vi "Arbitrary Monitor Multigraph.vi"() -> ()   [LabVIEW 2022 SP3]
uses:
  <instrlib>/tio-labview/TIO Library/TIO Stream Open.vi
  <instrlib>/tio-labview/TIO Library/TIO RPC Send REQuest.vi
  <instrlib>/tio-labview/TIO Library/TIO RPC Parse Reply.vi
  <instrlib>/tio-labview/TIO Library/TIO RPC Parse Reply Error.vi
  <instrlib>/tio-labview/TIO Library/TIO Data Stream Parse timebase Info.vi
  <instrlib>/tio-labview/TIO Library/TIO Data Stream Parse pstream Info.vi
  <instrlib>/tio-labview/TIO Library/TIO Data Stream Parse dstream Info.vi
  <vilib>/Utility/High Resolution Relative Seconds.vi
  <instrlib>/tio-labview/TIO Library/TIO Serial Port Name Search.vi
  <instrlib>/tio-labview/TIO Library/TIO Stream Write.vi
  <instrlib>/tio-labview/TIO Library/TIO RPC Form Request.vi
  <instrlib>/tio-labview/TIO Library/TIO SLIP Serial Write.vi
  <instrlib>/tio-labview/TIO Library/TIO Form Packet.vi
  <instrlib>/tio-labview/TIO Library/TIO SLIP Encode.vi
  <instrlib>/tio-labview/TIO Library/TIO Serial Checksum CRC32.vi
  <vilib>/Utility/tcp.llb/UDP Multicast Open.vi
  <vilib>/Utility/tcp.llb/UDP Multicast Read-Write Open.vi
  <instrlib>/tio-labview/TIO Library/TIO Serial Port Discovery.vi
  <vilib>/Instr/_visa.llb/VISA Configure Serial Port (Instr).vi
  <instrlib>/tio-labview/TIO Library/TIO RPC Blocking.vi
  <instrlib>/tio-labview/TIO Library/TIO Stream Read Non-blocking.vi
  <instrlib>/tio-labview/TIO Library/TIO RPC Send Heartbeat.vi
  <vilib>/Utility/file.llb/Write Delimited Spreadsheet (DBL).vi
panel:
  in  "Log":bool
  in  "File":path
  in  "String":string="gps"
  in  "Reset":bool
  in  "URL":refnum<visa-resource-name>="tcp://localhost"
  in  "Quit":bool
  in  "Duration":dbl[unit]=1000.0
  out "X":T1(graph)
  out "Y":T1(graph)
  out "Z":T1(graph)
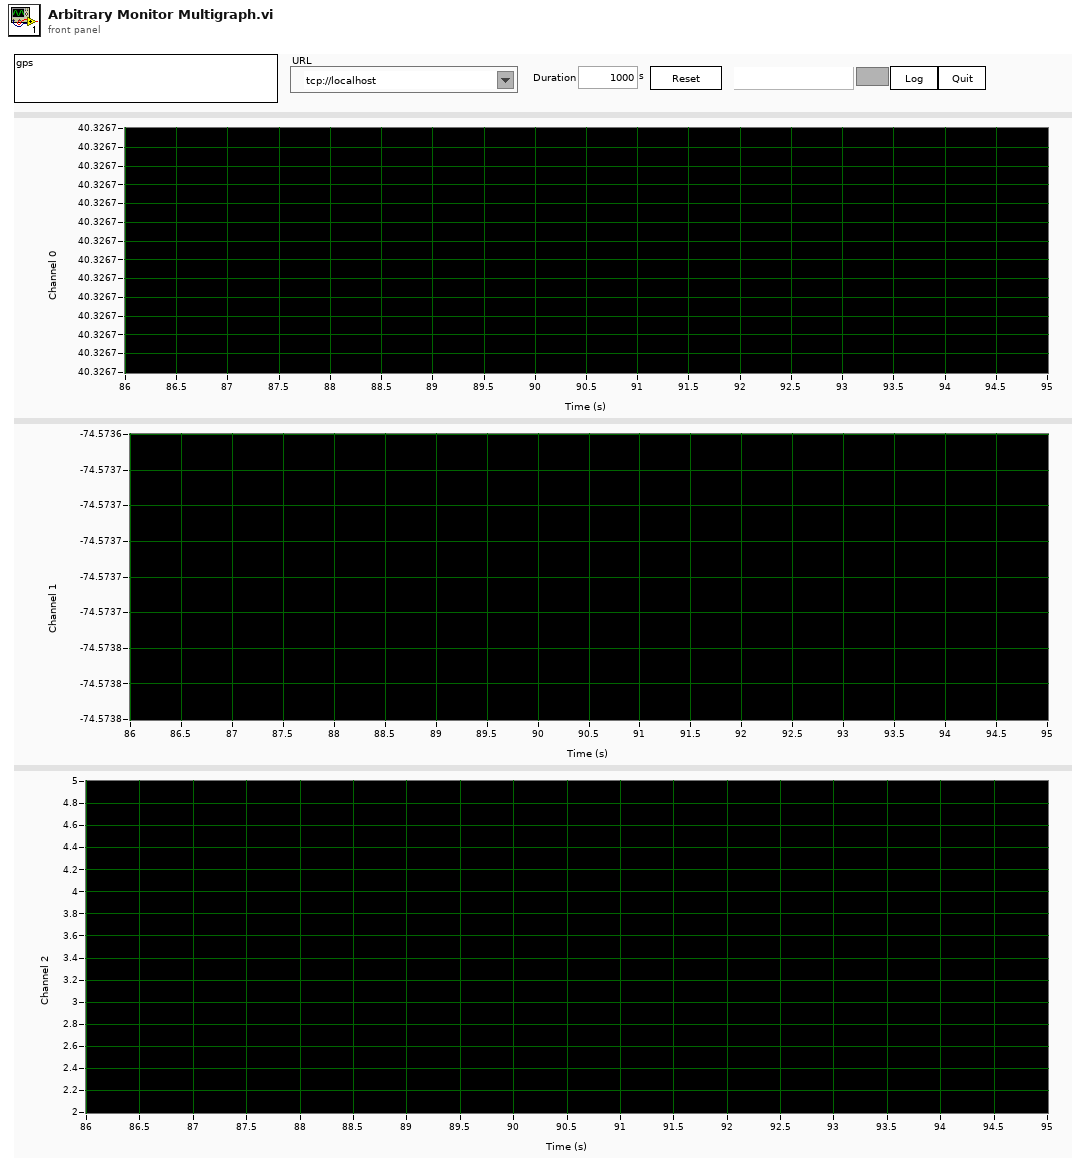
[diagram p1: front panel]
types:
  T1 = cluster{"start":dbl, "dt":dbl, "Timeseries":dbl[]}
  T2 = cluster{"TS Connection":cluster{"Type":enum16{"Serial", "TCP", "UDP", "mUDP"}, "URL":refnum<visa-resource-name>, "TO":u32, "Addr":u32, "Port":i32, "TCP":refnum<k5>, "UDP":refnum<k16>, "Route":string}, "REQ":refnum<queue>, "REP":refnum<queue>}
  T3 = cluster{"start":dbl, "dt":dbl, "Timeseries":sgl[][]}
  T4 = cluster{"Awaiting REP":bool, "REQ ID":u32, "streams in":cluster{"id":u16, "timebase id":u16, "period":u32, "offset":u32, "sample number":u64, "total components":u16, "flags":u16, "components":cluster{"source id":u16, "flags":u16, "period":u32, "offset":u32}[]}[], "sources":cluster{"id":u16, "timebase_id":u16, "period":u32, "offset":u32, "fmt":i32, "flags":u16, "channels":u16, "type":u8, "name":string, "column names":string[], "title":string, "units":string}[], "timebases":cluster{"id":u16, "source":u8, "epoch":u8, "start time":u64, "period numerator (µs)":u32, "period denominator (µs)":u32, "flags":u32, "stability":sgl, "source id":string}[]}
  T5 = cluster{"stream ID":u16, "Sample Number":u32, "Raw Data":string}
  T6 = cluster{"TC Connection":cluster{"Type":enum16{"Serial", "TCP", "UDP", "mUDP"}, "URL":refnum<visa-resource-name>, "TO":u32, "Addr":u32, "Port":i32, "TCP":refnum<k5>, "UDP":refnum<k16>, "Route":string}, "REQ":refnum<queue>, "REP":refnum<queue>}
  T7 = cluster{"start":dbl, "dt":dbl, "Timeseries":dbl[][]}
  T8 = cluster{"Name":string, "Waveform":cluster{"start":dbl, "dt":dbl, "Timeseries":dbl[][]}}[]
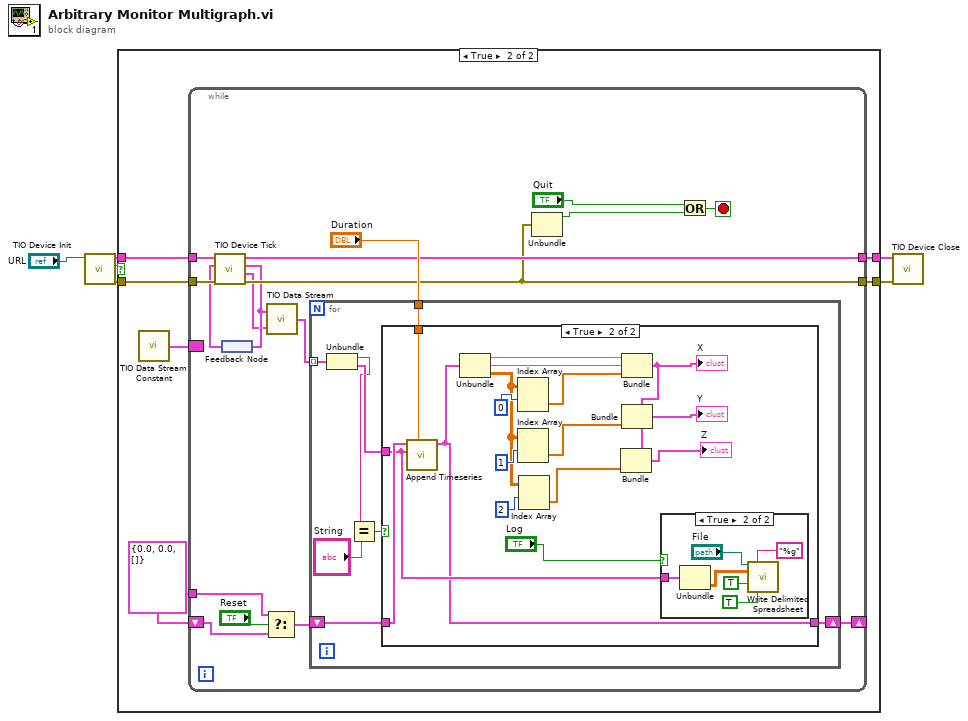
[diagram p0: block diagram]
diagram:
  n1 = call <instrlib>:"TIO Device Init.vi"("URL"="URL") -> ("error out"=w5:errorcluster, "ID Verified"=w3:bool, "TIO"=w6:T2)  [unwired: 6 in, 2 out]
  n2 = case shown="True" w3 {
    tunnel: w6 -> [w8 w10]
    tunnel: w5 -> [w7 w9]
    tunnel: [w7 w12] -> w2
    tunnel: [w8 w11] -> w1
    frame False {
    }
    frame True {
      w13 = T3 {"start"=0.0, "dt"=0.0, "Timeseries"=[]}
      n3 = call <instrlib>:"TIO Data Stream Constant.vi"() -> ("TIO State"=w14:T4)
      n4 = while {
        tunnel: w10 -> [w31]
        tunnel: w9 -> [w30]
        shift-right: [w28] -> _
        shift-left: w13 -> [w26]
        tunnel: [w21] -> w12
        border: w14 -> [_]
        tunnel: w13 -> [w24]
        tunnel: [w22] -> w11
        stop <- w18 stop-if-true
        n5 = feedback #1() -> (w27:T4)
        n6 = call <instrlib>:"TIO Device Tick.vi"("Error in"=w30, "TIO State"=w27, "TIO"=w31) -> ("Error out"=w21:errorcluster, "Data Out"=w15:T5, "TIO State"=w17:T4, "TIO"=w22:T6)  [unwired: 5 in]
        n7 = feedback-in #1(w17) -> ()
        n8 = Select(t=w24, s="Reset", f=w26) -> (s? t:f=w25:T7)
        n9 = call <instrlib>:"TIO Data Stream.vi"("Raw Data"=w15, "TIO State"=w17) -> ("Data Out"=w16:T8)
        n10 = for {
          tunnel: "Duration" -> [w39]
          tunnel: w16 -> [w36] mode=indexing
          shift-right: [w38] -> w28
          shift-left: w25 -> [w37]
          n11 = Unbundle(w36) -> ("Name"=w33:string, "Waveform"=w35:T7)
          n12 = Equal?(x=w33, y="String") -> (x = y?=w32:bool)
          n13 = case shown="True" w32 {
            tunnel: w39 -> [_ w57]
            tunnel: w35 -> [_ w55]
            tunnel: [w40 w53] -> w38
            tunnel: w37 -> [w40 w56]
            frame False {
            }
            frame True {
              n14 = call <instrlib>:"Append Timeseries.vi"("Duration"=w57, "In New"=w55, "In Old"=w56) -> ("Appended"=w53:T7)  [unwired: 8 in]
              n15 = Unbundle(w53) -> ("start"=w52:dbl, "dt"=w51:dbl, "Timeseries"=w44:dbl[][])
              n16 = Index Array(array=w44, index (row)=0 ("disabled index (col)")) -> (element=w50:dbl[])  [unwired: 1 in]
              n17 = Index Array(array=w44, index (row)=1 ("disabled index (col)")) -> (element=w49:dbl[])  [unwired: 1 in]
              n18 = Index Array(array=w44, index (row)=2 ("disabled index (col)")) -> (element=w43:dbl[])  [unwired: 1 in]
              n19 = Bundle("start"=w52, "dt"=w51, "Timeseries"=w50) -> (w42:T1)  [unwired: 1 in]
              "X" <- w42
              n20 = Bundle(cluster=w42, "Timeseries"=w43) -> (→"Z":T1)  [unwired: 2 in]
              n21 = Bundle(cluster=w42, "Timeseries"=w49) -> (→"Y":T1)  [unwired: 2 in]
              n22 = case shown="True" "Log" {
                tunnel: w55 -> [_ w60]
                frame False {
                }
                frame True {
                  n23 = Unbundle(w60) -> ("Timeseries"=w59:dbl[][])  [unwired: 2 out]
                  n24 = call-poly <vilib>:"Write Delimited Spreadsheet.vi"("file path (dialog if empty)"="File", "format (%.3f)"="%g", "2D data"=w59, "append to file? (new file:F)"=TRUE ("append to file? (F)"), "transpose? (no:F)"=TRUE ("transpose? (F)")) -> ()  [unwired: 9 in, 2 out]
                }
              }
            }
          }
        }
        n25 = Unbundle(w21) -> ("status"=w19:bool)  [unwired: 2 out]
        n26 = Or(x="Quit", y=w19) -> (x .or. y?=w18:bool)
      }
    }
  }
  n27 = call <instrlib>:"TIO Device Close.vi"("Error in"=w2, "TIO"=w1) -> ()  [unwired: 10 in]
